vi "Is Null.vi"(11 "Type in":refnum<class "Type.lvclass">) -> (2 "NULL":bool)   [LabVIEW 2020, in "Conditu2.lvlib" / "Columns.lvlib" / "Type.lvclass"]
uses:
  Type.lvclass
  Type.lvclass/Type.ctl
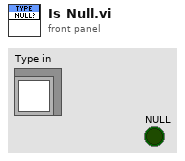
[diagram p1: front panel]
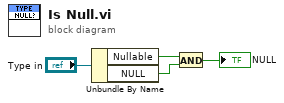
[diagram p0: block diagram]
diagram:
  n1 = Unbundle By Name("Type in") -> ("Nullable"=w3:bool, "NULL"=w2:bool)
  n2 = And(x=w3, y=w2) -> (x .and. y?=→"NULL":bool)
